vi "Write TOC [ ].vi"(0 "PDF Report Class in":refnum<class "PDF Report Class.lvclass">, 7 "TOC [ ]":T1[](array[typedef]), 11 "error in (no error)":errorcluster) -> (4 "PDF Report Class out":refnum<class "PDF Report Class.lvclass">, 15 "error out":errorcluster)   [LabVIEW 2019, in "PDF Report Class.lvclass"]
uses:
  <userlib>/Exaprom PDF/LV Class/PDF Report Class/PDF Report Class.lvclass
  <userlib>/Exaprom PDF/Controls/Chapter Controls/TOC Line.ctl
  <userlib>/Exaprom PDF/Controls/Text Controls/Unicode/Type and run direction.ctl
  <userlib>/Exaprom PDF/LV Class/PDF Report Class/PDF Report Class.lvclass/PDF Report Class.ctl
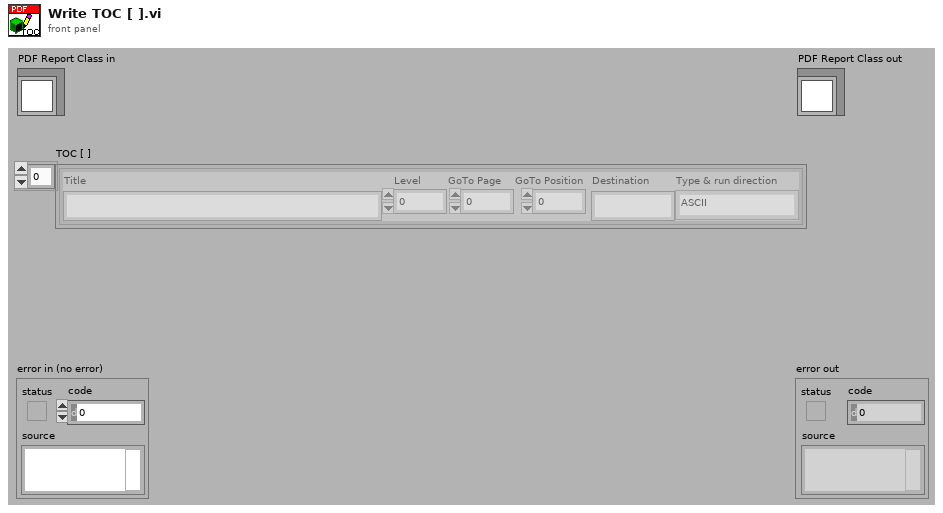
[diagram p1: front panel]
types:
  T1 = typedef "TOC Line.ctl" = cluster{"Title":string, "Level":u16, "GoTo Page":u16, "GoTo Position":u16, "Destination":string, "Type & run direction":T2}
  T2 = typedef "Type and run direction.ctl" = enum16{"Select", "ASCII", "UTF-16", "UTF-16 (default)", "UTF-16 (LTR)", "UTF-16 (RTL)"}
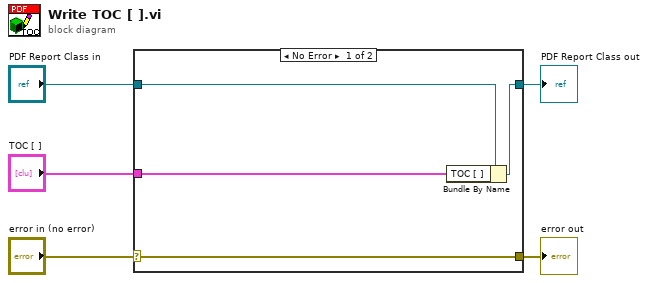
[diagram p0: block diagram]
diagram:
  n1 = case shown="No Error" "error in (no error)" {
    selector: "error in (no error)" -> [w9 w10]
    tunnel: [w9 w10] -> w4
    tunnel: [w7 w11] -> w2
    tunnel: "PDF Report Class in" -> [w8 w11]
    tunnel: "TOC [ ]" -> [w6 _]
    frame No Error {
      n2 = Bundle By Name(cluster=w8, "TOC [ ]"=w6) -> (w7:refnum<class "PDF Report Class.lvclass">)
    }
    frame Error {
    }
  }
  "error out" <- w4
  "PDF Report Class out" <- w2
